vi "QI.vi"(8 "error in (no error)":errorcluster caption="错误输入（无错误）", 10 "图像信号输入":dbl[][](array[numeric])) -> (0 "error out":errorcluster caption="错误输出", 1 "Y_c":dbl, 2 "X_c":dbl)   [LabVIEW 2013]
doc: "使用该模板构建标准状态机设计模式。各状态执行代码并决定转移状态。将该设计模式与根据用户动作响应而执行代码的用户界面事件处理器模式相比较。同时将该设计模式与每段消息处理代码可以将零至多个新消息加入队列的队列消息处理器模式相比较。\n注：该模板的设计未遵守最新NI推荐的编程风格。请通过“创建项目”对话框（而不要采用该模板），创建基于项目的标准状态机模式的完整实现。"
uses:
  QI state.ctl
panel:
  in  "传递变量":T1
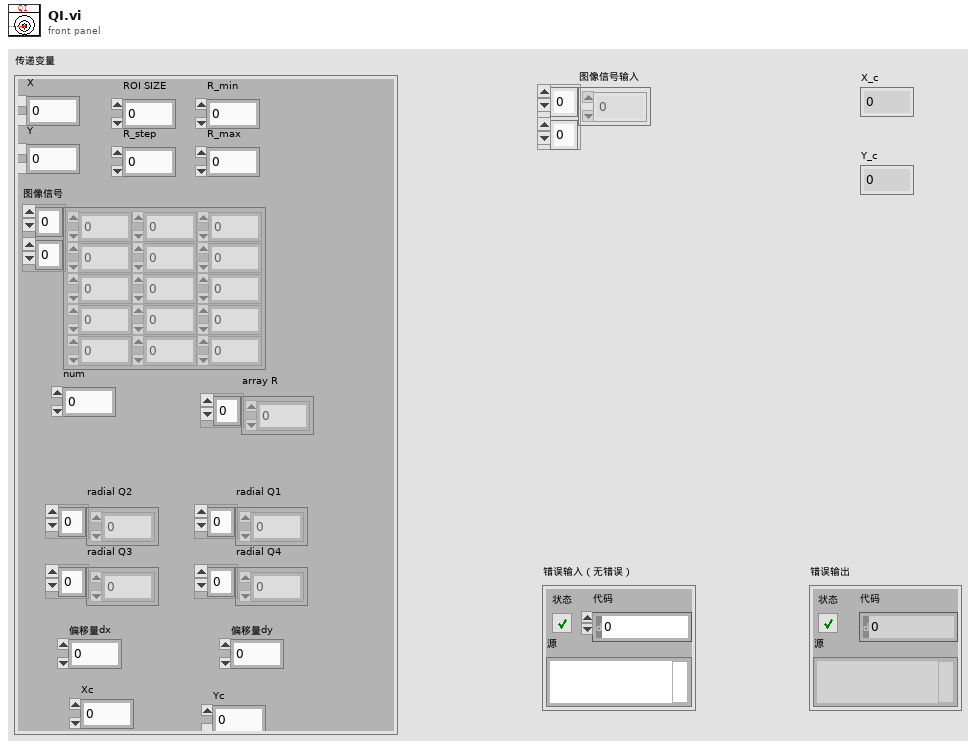
[diagram p1: front panel]
types:
  T1 = cluster{"X":dbl, "Y":dbl, "图像信号":dbl[][], "ROI SIZE":i32, "R_step":dbl, "R_min":dbl, "R_max":dbl, "num":dbl, "array R":dbl[], "radial Q1":dbl[], "radial Q2":dbl[], "radial Q3":dbl[], "radial Q4":dbl[], "偏移量dx":dbl, "偏移量dy":dbl, "Xc":dbl, "Yc":dbl}
  T2 = typedef "QI state.ctl" = enum16{"初始化", "图心估计", "径向分布", "相关性分析XY", "修正XY"}
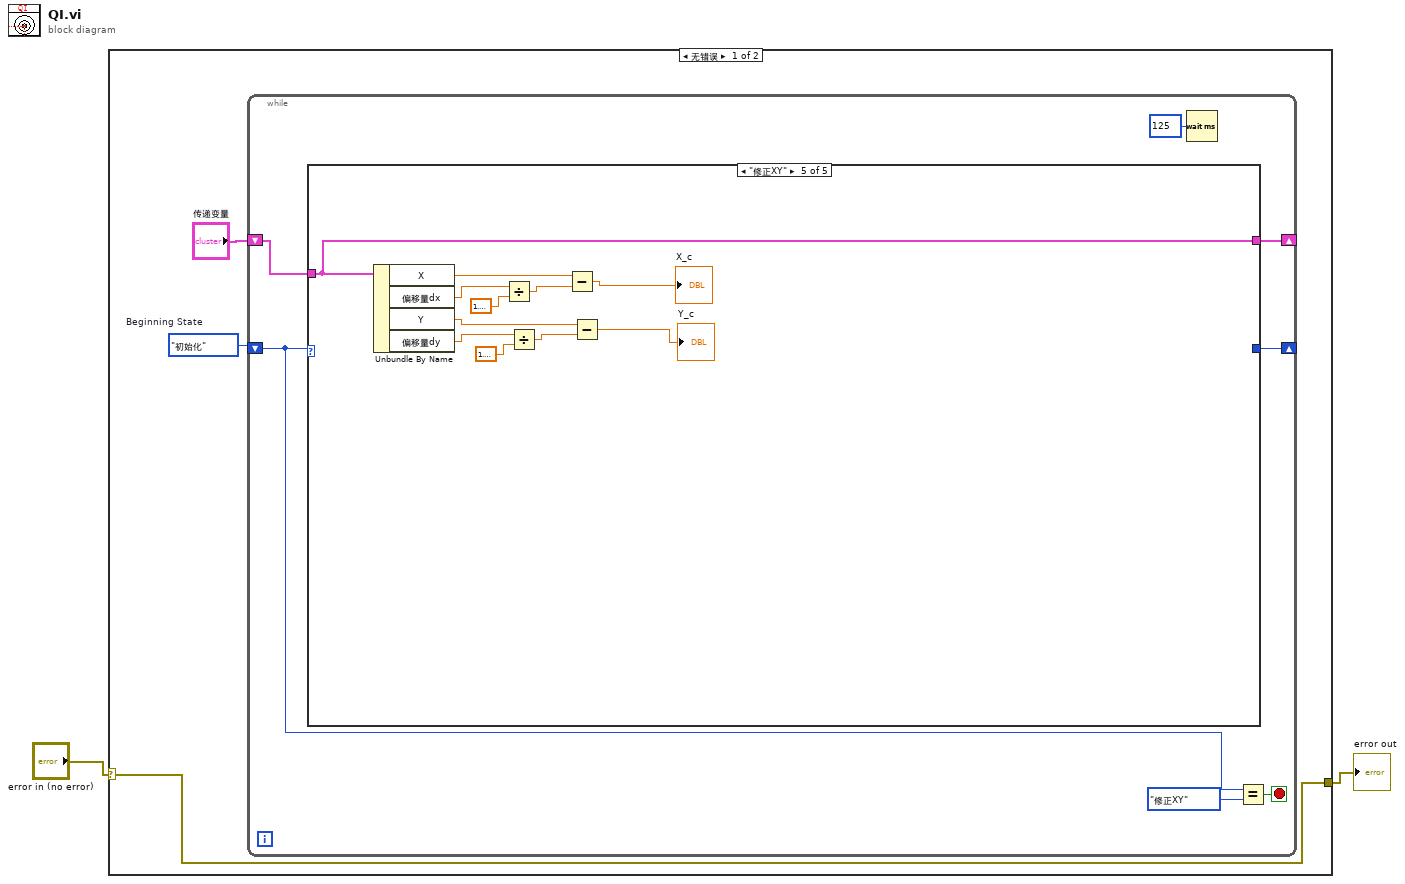
[diagram p0: block diagram]
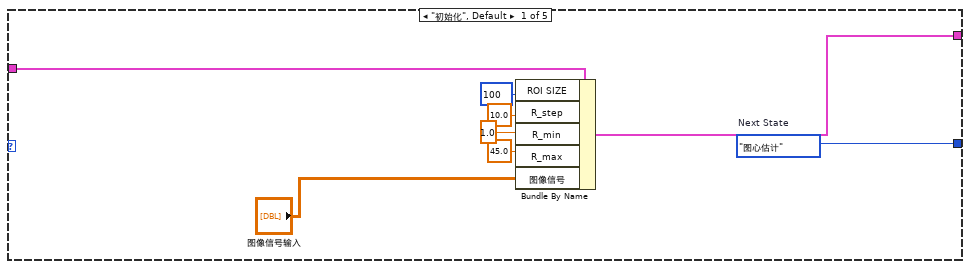
[diagram p2: hidden frame]
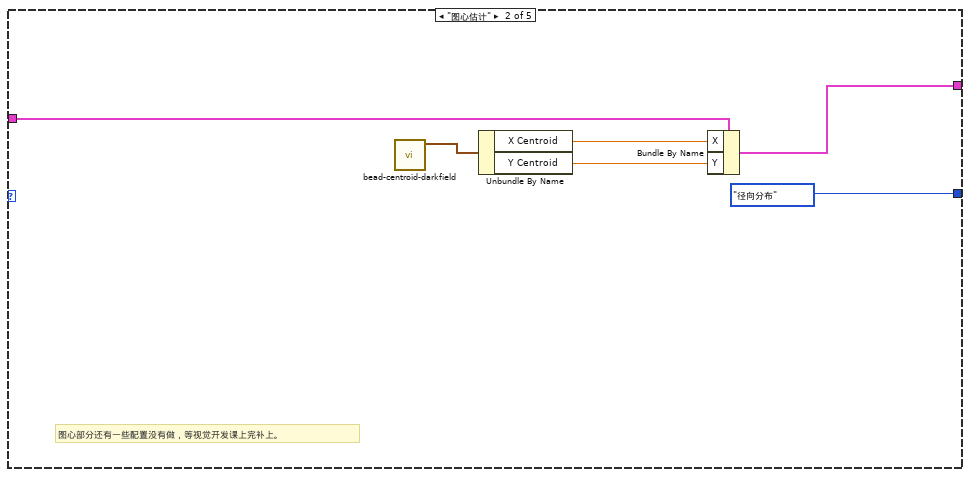
[diagram p3: hidden frame]
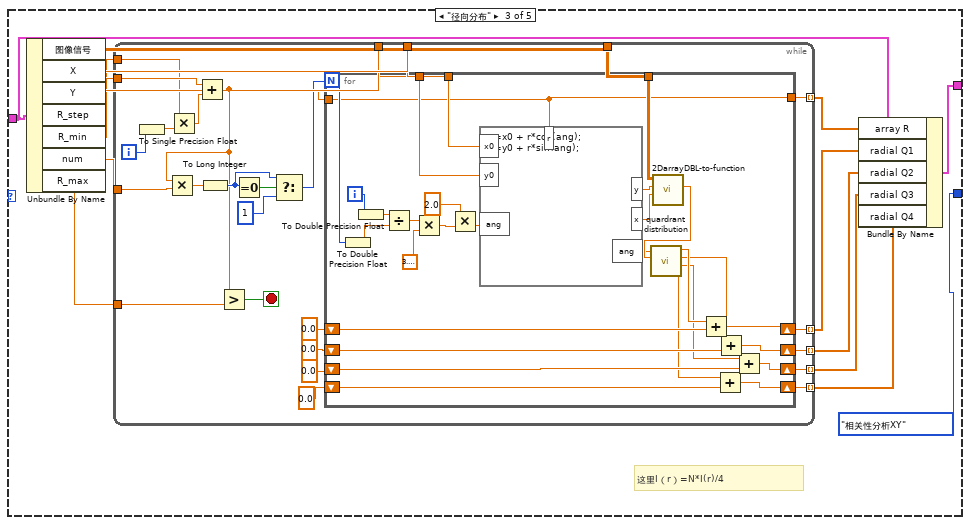
[diagram p4: hidden frame]
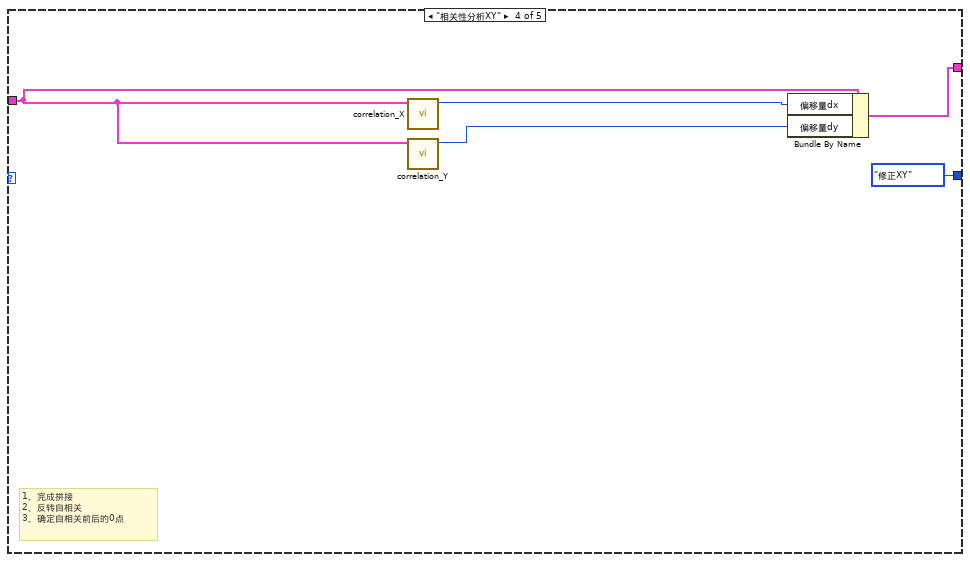
[diagram p5: hidden frame]
diagram:
  n1 = case shown="无错误" "error in (no error)" {
    selector: "error in (no error)" -> [w3 w113]
    tunnel: [w3 w113] -> w1
    frame No Error {
      w5 = QI_state."初始化"  # Beginning State
      n2 = while {
        shift-right: [w9] -> _
        shift-left: w5 -> [w10]
        shift-right: [w6] -> _
        shift-left: "传递变量" -> [w7]
        stop <- w12 stop-if-true
        n3 = case shown="\"修正XY\"" w10 {
          tunnel: [w20 QI_state."径向分布" ("Next State") QI_state."相关性分析XY" ("Next State") QI_state."修正XY" ("Next State") _] -> w9
          tunnel: w7 -> [w19 w24 w32 w98 w108]
          tunnel: [w17 w23 w33 w100 w108] -> w6
          frame "初始化", Default {
            w20 = QI_state."图心估计"  # Next State
            n4 = Bundle By Name(cluster=w19, "ROI SIZE"=100, "R_step"=10.0, "R_min"=1.0, "R_max"=45.0, "图像信号"="图像信号输入") -> (w17:T1)
          }
          frame "图心估计" {
            # "图心部分还有一些配置没有做，等视觉开发课上完补上。"
            n5 = call "bead-centroid-darkfield.vi"() -> ("Centroid"=w25:cluster{"X Centroid":sgl, "Y Centroid":sgl})  [unwired: 8 in, 3 out]
            n6 = Unbundle By Name(w25) -> ("X Centroid"=w22:sgl, "Y Centroid"=w21:sgl)
            n7 = Bundle By Name(cluster=w24, "X"=w22, "Y"=w21) -> (w23:T1)
          }
          frame "径向分布" {
            # "这里I（r）=N*I(r)/4"
            n8 = Unbundle By Name(w32) -> ("图像信号"=w39:dbl[][], "X"=w41:dbl, "Y"=w40:dbl, "R_step"=w37:dbl, "R_min"=w38:dbl, "num"=w36:dbl, "R_max"=w35:dbl)
            n9 = while {
              tunnel: w41 -> [w67]
              tunnel: w40 -> [w66]
              tunnel: w39 -> [w65]
              tunnel: w38 -> [w56]
              tunnel: w37 -> [w55]
              tunnel: w36 -> [w54]
              tunnel: w35 -> [w53]
              tunnel: [w46] -> w30 mode=indexing
              tunnel: [w45] -> w29 mode=indexing
              tunnel: [w44] -> w28 mode=indexing
              tunnel: [w43] -> w27 mode=indexing
              tunnel: [w42] -> w31 mode=indexing
              i -> [w57]
              stop <- w51 stop-if-true
              n10 = To Single Precision Float(number=w57) -> (single precision float=w61:sgl)
              n11 = Multiply(x=w55, y=w61) -> (x*y=w59:dbl)
              n12 = Add(x=w56, y=w59) -> (x+y=w52:dbl)
              n13 = Multiply(x=w52, y=w54) -> (x*y=w60:dbl)
              n14 = To Long Integer(number=w60) -> (32bit integer=w58:i32)
              n15 = Greater?(x=w52, y=w53) -> (0:w51:bool)
              n16 = Equal To 0?(x=w58) -> (x = 0?=w64:bool)
              n17 = Select(t=w58, s=w64, f=1) -> (s? t:f=w62:i32)
              n18 = for {
                N: w62 -> [w85]
                tunnel: w67 -> [w91]
                tunnel: w66 -> [w90]
                tunnel: w65 -> [w87]
                tunnel: w52 -> [w68]
                shift-right: [w77] -> w46
                shift-left: 0.0 -> [w79]
                shift-right: [w76] -> w45
                shift-left: 0.0 -> [w72]
                shift-right: [w80] -> w44
                shift-left: 0.0 -> [w73]
                shift-right: [w75] -> w43
                shift-left: 0.0 -> [w74]
                tunnel: [w68] -> w42
                i -> [w86]
                n19 = To Double Precision Float(number=w85) -> (double precision float=w92:dbl)
                n20 = To Double Precision Float(number=w86) -> (double precision float=w93:dbl)
                n21 = Divide(x=w93, y=w92) -> (x/y=w96:dbl)
                n22 = Multiply(x=w96, y=3.141592653589793) -> (x*y=w95:dbl)
                n23 = Multiply(x=2.0, y=w95) -> (x*y=w84:dbl)
                n24 = formula code="x=x0 + r*cos(ang);\ny=y0 + r*sin(ang);"("x0"=w91, "y0"=w90, "ang"=w84, "r"=w68) -> ("x"=w89:dbl, "y"=w88:dbl, "ang"=w81:dbl)
                n25 = call "2DarrayDBL-to-function.vi"("X"=w89, "Y"=w88, "2D array"=w87) -> ("f(x,y)"=w82:dbl)  [unwired: 6 in, 2 out]
                n26 = call "quardrant distribution.vi"("angle"=w81, "input radial point"=w82) -> ("quardrant 4"=w69:dbl, "quardrant 3"=w70:dbl, "quardrant 2"=w71:dbl, "quardrant 1"=w78:dbl)  [unwired: 6 in]
                n27 = Add(x=w78, y=w79) -> (x+y=w77:dbl)
                n28 = Add(x=w69, y=w74) -> (x+y=w75:dbl)
                n29 = Add(x=w71, y=w72) -> (x+y=w76:dbl)
                n30 = Add(x=w70, y=w73) -> (x+y=w80:dbl)
              }
            }
            n31 = Bundle By Name(cluster=w32, "array R"=w31, "radial Q1"=w30, "radial Q2"=w29, "radial Q3"=w28, "radial Q4"=w27) -> (w33:T1)
          }
          frame "相关性分析XY" {
            # "1、完成拼接\n2、反转自相关\n3、确定自相关前后的0点"
            n32 = call "correlation_X.vi"("传递变量"=w98) -> ("数值"=w101:i32)  [unwired: 10 in]
            n33 = call "correlation_Y.vi"("传递变量"=w98) -> ("数值"=w97:i32)  [unwired: 10 in]
            n34 = Bundle By Name(cluster=w98, "偏移量dx"=w101, "偏移量dy"=w97) -> (w100:T1)
          }
          frame "修正XY" {
            n35 = Unbundle By Name(w108) -> ("X"=w110:dbl, "偏移量dx"=w111:dbl, "Y"=w105:dbl, "偏移量dy"=w104:dbl)
            n36 = Divide(x=w111, y=1.5707963267948966) -> (x/y=w109:dbl)
            n37 = Divide(x=w104, y=1.5707963267948966) -> (x/y=w107:dbl)
            n38 = Subtract(x=w110, y=w109) -> (x-y=→"X_c":dbl)
            n39 = Subtract(x=w105, y=w107) -> (x-y=→"Y_c":dbl)
          }
        }
        n40 = Wait (ms)(milliseconds to wait=u32 125) -> ()  [unwired: 1 out]
        n41 = Equal?(x=w10, y=QI_state."修正XY" ("States")) -> (x = y?=w12:bool)
      }
    }
    frame Error {
    }
  }
  "error out" <- w1
